vi "XXPathPlanner_Path_RePlan_Worker3.vi"(4 "StartingPoseTranslation":T1 {"Y" format="%14.3f"; "X" format="%14.3f"}, 5 "in PathPlannerPath":T2={"Reversed"=FALSE, "RotationTargets"=[], "ConstraintZones"=[], "EventMarkers"=[], "GlobalConstraints"={"MaxVelocityMps;"=0.0, "MaxAccelerationMpsSq;"=0.0, "MaxAngularVelRadPsEc;"=0.0, "MaxAngularAccRadPSecSq"=0.0, "Exists"=FALSE, "Unlimited"=FALSE, "NominalVoltageVolts"=12.0}, "GoalEndState"={"VelocityMPS"=0.0, "Rotation"={"VALUE"=0.0, "COS"=0.0, "SIN"=0.0}}, "AllPoints"=[], "Name"="", "Waypoints"=[], "PointTowardsZones"=[], "IdealStartingState"={"VelocityMPS"=0.0, "Rotation"={"VALUE"=0.0, "COS"=0.0, "SIN"=0.0}}, "IsChoreoPath"=FALSE, "PreventFlipping"=FALSE} {"IdealStartingState"."Rotation"."SIN" format="%13.4f"; "IdealStartingState"."Rotation"."COS" format="%13.4f"; "IdealStartingState"."Rotation"."VALUE" format="%13.4f"; "PointTowardsZones"."TargetPosition"."Y" format="%14.3f"; "PointTowardsZones"."TargetPosition"."X" format="%14.3f"; "PointTowardsZones"."RotationOffset"."SIN" format="%13.4f"; "PointTowardsZones"."RotationOffset"."COS" format="%13.4f"; "PointTowardsZones"."RotationOffset"."VALUE" format="%13.4f"; "Waypoints"."nextControl"."Y" format="%14.3f"; "Waypoints"."nextControl"."X" format="%14.3f"; "Waypoints"."anchor"."Y" format="%14.3f"; "Waypoints"."anchor"."X" format="%14.3f"; "Waypoints"."prevControl"."Y" format="%14.3f"; "Waypoints"."prevControl"."X" format="%14.3f"; "AllPoints"."RotationTarget"."rotation"."SIN" format="%13.4f"; "AllPoints"."RotationTarget"."rotation"."COS" format="%13.4f"; "AllPoints"."RotationTarget"."rotation"."VALUE" format="%13.4f"; "AllPoints"."Position"."Y" format="%14.3f"; "AllPoints"."Position"."X" format="%14.3f"; "GoalEndState"."Rotation"."SIN" format="%13.4f"; "GoalEndState"."Rotation"."COS" format="%13.4f"; "GoalEndState"."Rotation"."VALUE" format="%13.4f"; "RotationTargets"."rotation"."SIN" format="%13.4f"; "RotationTargets"."rotation"."COS" format="%13.4f"; "RotationTargets"."rotation"."VALUE" format="%13.4f"}, 6 "robotNextCtrl":T1 {"Y" format="%14.3f"; "X" format="%14.3f"}, 7 "NumPtsMinusOne":i32, 8 "ClosestPointIdx":i32, 9 "robotNextCtrl_NULL":bool, 11 "ClosestDist":dbl) -> (2 "Error":bool, 3 "Replanned Path":T2={"Reversed"=FALSE, "RotationTargets"=[], "ConstraintZones"=[], "EventMarkers"=[], "GlobalConstraints"={"MaxVelocityMps;"=0.0, "MaxAccelerationMpsSq;"=0.0, "MaxAngularVelRadPsEc;"=0.0, "MaxAngularAccRadPSecSq"=0.0, "Exists"=FALSE, "Unlimited"=FALSE, "NominalVoltageVolts"=12.0}, "GoalEndState"={"VelocityMPS"=0.0, "Rotation"={"VALUE"=0.0, "COS"=0.0, "SIN"=0.0}}, "AllPoints"=[], "Name"="", "Waypoints"=[], "PointTowardsZones"=[], "IdealStartingState"={"VelocityMPS"=0.0, "Rotation"={"VALUE"=0.0, "COS"=0.0, "SIN"=0.0}}, "IsChoreoPath"=FALSE, "PreventFlipping"=FALSE} {"IdealStartingState"."Rotation"."SIN" format="%13.4f"; "IdealStartingState"."Rotation"."COS" format="%13.4f"; "IdealStartingState"."Rotation"."VALUE" format="%13.4f"; "PointTowardsZones"."TargetPosition"."Y" format="%14.3f"; "PointTowardsZones"."TargetPosition"."X" format="%14.3f"; "PointTowardsZones"."RotationOffset"."SIN" format="%13.4f"; "PointTowardsZones"."RotationOffset"."COS" format="%13.4f"; "PointTowardsZones"."RotationOffset"."VALUE" format="%13.4f"; "Waypoints"."nextControl"."Y" format="%14.3f"; "Waypoints"."nextControl"."X" format="%14.3f"; "Waypoints"."anchor"."Y" format="%14.3f"; "Waypoints"."anchor"."X" format="%14.3f"; "Waypoints"."prevControl"."Y" format="%14.3f"; "Waypoints"."prevControl"."X" format="%14.3f"; "AllPoints"."RotationTarget"."rotation"."SIN" format="%13.4f"; "AllPoints"."RotationTarget"."rotation"."COS" format="%13.4f"; "AllPoints"."RotationTarget"."rotation"."VALUE" format="%13.4f"; "AllPoints"."Position"."Y" format="%14.3f"; "AllPoints"."Position"."X" format="%14.3f"; "GoalEndState"."Rotation"."SIN" format="%13.4f"; "GoalEndState"."Rotation"."COS" format="%13.4f"; "GoalEndState"."Rotation"."VALUE" format="%13.4f"; "RotationTargets"."rotation"."SIN" format="%13.4f"; "RotationTargets"."rotation"."COS" format="%13.4f"; "RotationTargets"."rotation"."VALUE" format="%13.4f"})   [LabVIEW 2019]
doc: "Replan path worker 3\n\nInternal routine. Not for end user use."
uses:
  PathPlanner24.lvlib
  <vilib>/Rock Robotics/WPI/ThirdParty/JAS_Junk/TrajLib/Trajectory_Library.lvlib
  <vilib>/Rock Robotics/WPI/ThirdParty/JAS_Junk/TrajLib/TypeDef/TRANSLATION2D.ctl
  <vilib>/Rock Robotics/WPI/ThirdParty/JAS_Junk/TrajLib/TypeDef/ROTATION2D.ctl
  TypeDef/PathPlannerRotationTarget.ctl
  TypeDef/PathPlannerPathConstraints.ctl
  TypeDef/PathPlannerConstraintsZone.ctl
  ENum/PathPlanner_CommandUtilType_ENUM.ctl
  TypeDef/PathPlannerCommandUtil.ctl
  TypeDef/PathPlannerEventMarker.ctl
  TypeDef/PathPlannerGoalEndState.ctl
  TypeDef/PathPlannerPathPoint.ctl
  TypeDef/PathPlannerPath.ctl
  TypeDef/PathPlannerWaypoint.ctl
  TypeDef/PathPlannerPointTowardsZone.ctl
  TypeDef/PathPlannerIdealStartingState.ctl
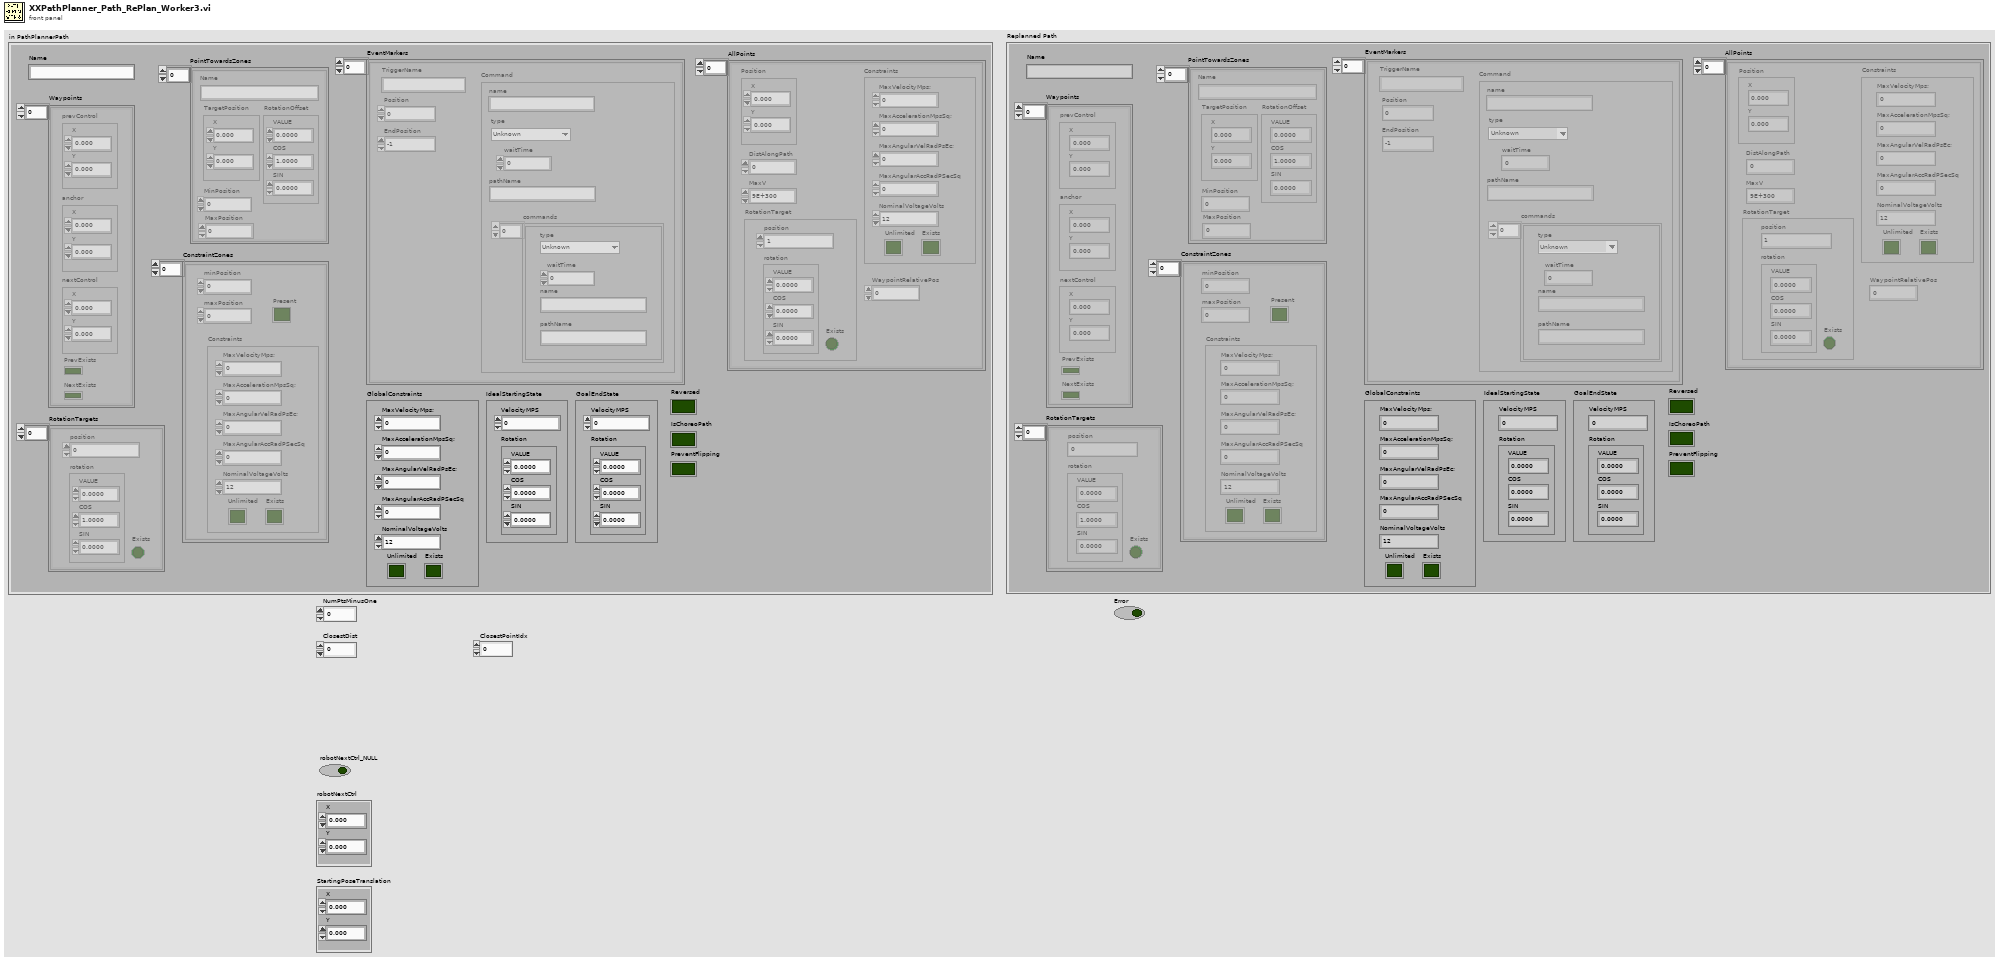
[diagram p1: front panel]
types:
  T1 = typedef "Trajectory_Library.lvlib/TRANSLATION2D.ctl" = cluster{"X":dbl, "Y":dbl}
  T2 = typedef "PathPlanner24.lvlib/PathPlannerPath.ctl" = cluster{"Reversed":bool, "RotationTargets":T3[], "ConstraintZones":T5[], "EventMarkers":T7[], "GlobalConstraints":T6, "GoalEndState":T10, "AllPoints":T11[], "Name":string, "Waypoints":T12[], "PointTowardsZones":T13[], "IdealStartingState":T14, "IsChoreoPath":bool, "PreventFlipping":bool}
  T3 = typedef "PathPlanner24.lvlib/PathPlannerRotationTarget.ctl" = cluster{"rotation":T4, "position":dbl, "Exists":bool}
  T4 = typedef "Trajectory_Library.lvlib/ROTATION2D.ctl" = cluster{"VALUE":dbl, "COS":dbl, "SIN":dbl}
  T5 = typedef "PathPlanner24.lvlib/PathPlannerConstraintsZone.ctl" = cluster{"minPosition":dbl, "maxPosition":dbl, "Constraints":T6, "Present":bool}
  T6 = typedef "PathPlanner24.lvlib/PathPlannerPathConstraints.ctl" = cluster{"MaxVelocityMps;":dbl, "MaxAccelerationMpsSq;":dbl, "MaxAngularVelRadPsEc;":dbl, "MaxAngularAccRadPSecSq":dbl, "Exists":bool, "Unlimited":bool, "NominalVoltageVolts":dbl}
  T7 = typedef "PathPlanner24.lvlib/PathPlannerEventMarker.ctl" = cluster{"Position":dbl, "Command":T8, "TriggerName":string, "EndPosition":dbl}
  T8 = typedef "PathPlanner24.lvlib/PathPlannerCommandUtil.ctl" = cluster{"waitTime":dbl, "name":string, "pathName":string, "commands":cluster{"type":T9, "waitTime":dbl, "name":string, "pathName":string}[], "type":T9}
  T9 = typedef "PathPlanner24.lvlib/PathPlanner_CommandUtilType_ENUM.ctl" = enum16{"Unknown", "Wait", "Named", "Path", "Sequential", "Parallel", "Race", "Deadline"}
  T10 = typedef "PathPlanner24.lvlib/PathPlannerGoalEndState.ctl" = cluster{"VelocityMPS":dbl, "Rotation":T4}
  T11 = typedef "PathPlanner24.lvlib/PathPlannerPathPoint.ctl" = cluster{"Position":T1, "DistAlongPath":dbl, "MaxV":dbl, "Constraints":T6, "RotationTarget":T3, "WaypointRelativePos":dbl}
  T12 = typedef "PathPlanner24.lvlib/PathPlannerWaypoint.ctl" = cluster{"prevControl":T1, "anchor":T1, "nextControl":T1, "PrevExists":bool, "NextExists":bool}
  T13 = typedef "PathPlanner24.lvlib/PathPlannerPointTowardsZone.ctl" = cluster{"RotationOffset":T4, "Name":string, "TargetPosition":T1, "MinPosition":dbl, "MaxPosition":dbl}
  T14 = typedef "PathPlanner24.lvlib/PathPlannerIdealStartingState.ctl" = cluster{"VelocityMPS":dbl, "Rotation":T4}
  T15 = typedef "PathPlannerPathSegment.ctl" = cluster{"SegmentPoints":T11[]}
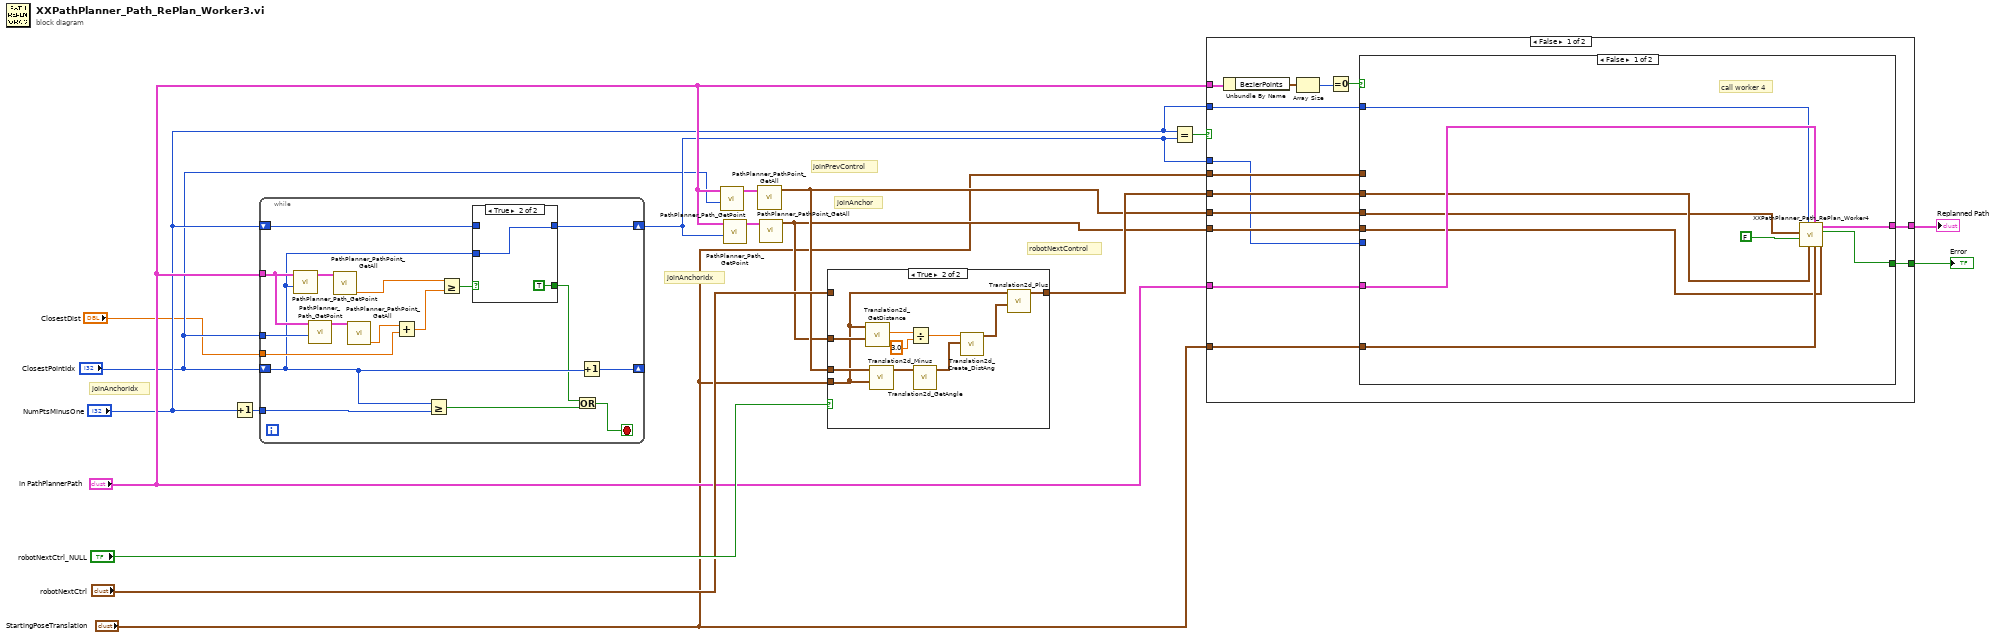
[diagram p0: block diagram]
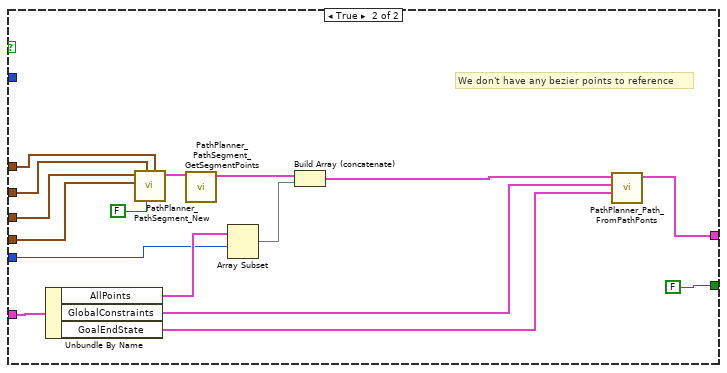
[diagram p2: hidden frame]
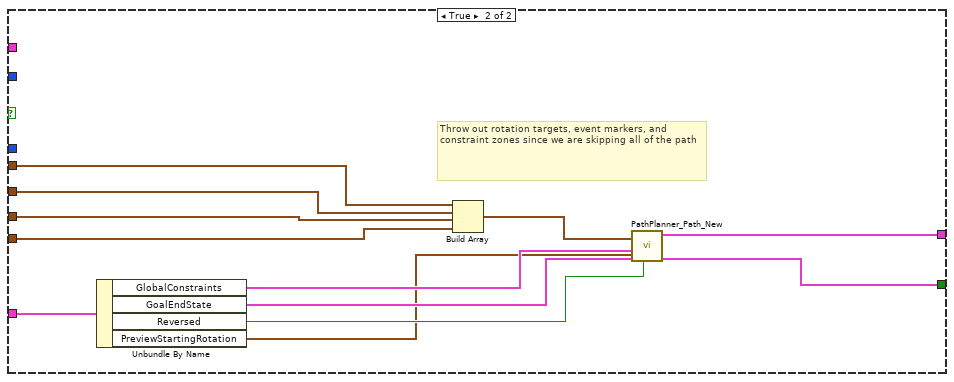
[diagram p3: hidden frame]
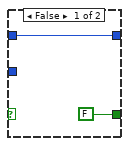
[diagram p5: hidden frame]
diagram:
  # "robotNextControl"
  # "joinAnchor"
  # "joinPrevControl"
  # "joinAnchorIdx"
  # "joinAnchorIdx"
  n1 = Increment(x="NumPtsMinusOne") -> (x+1=w17:i32)
  n2 = while {
    shift-right: [w33] -> _
    shift-left: "ClosestPointIdx" -> [w21]
    tunnel: w17 -> [w34]
    tunnel: "in PathPlannerPath" -> [w29]
    tunnel: "ClosestPointIdx" -> [w30]
    tunnel: "ClosestDist" -> [w27]
    shift-right: [w19] -> w5
    shift-left: "NumPtsMinusOne" -> [w20]
    stop <- w22 stop-if-true
    n3 = call "PathPlanner_Path_GetPoint.vi"("Index"=w21, "PathPlannerPath"=w29) -> ("Point"=w32:T11)  [unwired: 9 in]
    n4 = call "PathPlanner_Path_GetPoint.vi"("Index"=w30, "PathPlannerPath"=w29) -> ("Point"=w31:T11)  [unwired: 9 in]
    n5 = call "PathPlanner_PathPoint_GetAll.vi"("PathPlannerPoint"=w32) -> ("DistAlongPath"=w26:dbl)  [unwired: 5 in, 5 out]
    n6 = call "PathPlanner_PathPoint_GetAll.vi"("PathPlannerPoint"=w31) -> ("DistAlongPath"=w28:dbl)  [unwired: 5 in, 5 out]
    n7 = Add(x=w28, y=w27) -> (x+y=w25:dbl)
    n8 = Greater Or Equal?(x=w21, y=w34) -> (x >= y?=w23:bool)
    n9 = Greater Or Equal?(x=w26, y=w25) -> (x >= y?=w24:bool)
    n10 = case shown="True" w24 {
      tunnel: w21 -> [_ w38]
      tunnel: w20 -> [w36 _]
      tunnel: [w36 w38] -> w19
      tunnel: [FALSE TRUE] -> w18
      frame False {
      }
      frame True {
      }
    }
    n11 = Or(x=w18, y=w23) -> (x .or. y?=w22:bool)
    n12 = Increment(x=w21) -> (x+1=w33:i32)
  }
  n13 = call "PathPlanner_Path_GetPoint.vi"("Index"="ClosestPointIdx", "PathPlannerPath"="in PathPlannerPath") -> ("Point"=w16:T11)  [unwired: 9 in]
  n14 = call "PathPlanner_Path_GetPoint.vi"("Index"=w5, "PathPlannerPath"="in PathPlannerPath") -> ("Point"=w15:T11)  [unwired: 9 in]
  n15 = call "PathPlanner_PathPoint_GetAll.vi"("PathPlannerPoint"=w16) -> ("Position"=w10:T1)  [unwired: 5 in, 5 out]
  n16 = call "PathPlanner_PathPoint_GetAll.vi"("PathPlannerPoint"=w15) -> ("Position"=w9:T1)  [unwired: 5 in, 5 out]
  n17 = case shown="True" "robotNextCtrl_NULL" {
    tunnel: "robotNextCtrl" -> [w39 _]
    tunnel: [w39 w42] -> w11
    tunnel: w9 -> [_ w45]
    tunnel: w10 -> [_ w46]
    tunnel: "StartingPoseTranslation" -> [_ w44]
    frame False {
    }
    frame True {
      n18 = call <vilib>:"Translation2d_GetDistance.vi"("other Translation"=w45, "In Translation"=w44) -> ("Distance"=w48:dbl)  [unwired: 9 in]
      n19 = call <vilib>:"Translation2d_Minus.vi"("other Translation"=w44, "In Translation"=w46) -> ("Out Translation"=w49:T1)  [unwired: 9 in]
      n20 = Divide(x=w48, y=3.0) -> (x/y=w41:dbl)
      n21 = call <vilib>:"Translation2d_GetAngle.vi"("In Translation"=w49) -> ("Angle_Rotation2d"=w40:T4)  [unwired: 10 in]
      n22 = call <vilib>:"Translation2d_Create_DistAng.vi"("Angle"=w40, "Dist"=w41) -> ("TRANSLATION"=w43:T1)  [unwired: 9 in]
      n23 = call <vilib>:"Translation2d_Plus.vi"("other Translation"=w43, "In Translation"=w44) -> ("Out Translation"=w42:T1)  [unwired: 9 in]
    }
  }
  n24 = Equal?(x="NumPtsMinusOne", y=w5) -> (x = y?=w12:bool)
  n25 = case shown="False" w12 {
    tunnel: "StartingPoseTranslation" -> [w56 w100]
    tunnel: w11 -> [w55 w99]
    tunnel: w10 -> [w54 w98]
    tunnel: w9 -> [w53 w97]
    tunnel: "in PathPlannerPath" -> [w59 w95]
    tunnel: [w58 w90] -> w8
    tunnel: [w57 w89] -> w7
    tunnel: "in PathPlannerPath" -> [w63 _]
    tunnel: w5 -> [w52 _]
    tunnel: "NumPtsMinusOne" -> [w51 _]
    tunnel: "StartingPoseTranslation" -> [w50 _]
    frame False {
      n26 = Unbundle By Name(w63) -> ("BezierPoints"=w62:T1[])
      n27 = Array Size(array=w62) -> (size(s)=w61:i32)
      n28 = Equal To 0?(x=w61) -> (x = 0?=w60:bool)
      n29 = case shown="False" w60 {
        tunnel: w59 -> [w70 w88]
        tunnel: [w72 w74] -> w58
        tunnel: [w71 FALSE] -> w57
        tunnel: w56 -> [_ w87]
        tunnel: w55 -> [w67 w86]
        tunnel: w54 -> [w64 w85]
        tunnel: w53 -> [w65 w84]
        tunnel: w52 -> [_ w79]
        tunnel: w51 -> [w69 _]
        tunnel: w50 -> [w66 _]
        frame False {
          # "call worker 4"
          n30 = call "XXPathPlanner_Path_RePlan_Worker4.vi"("JoinAnchor"=w65, "StartingPoseTranslation"=w66, "in PathPlannerPath"=w70, "robotNextCtrl"=w67, "NumPtsMinusOne"=w69, "robotNextCtrl_NULL"=FALSE, "JoinPrevCtrl"=w64) -> ("Error"=w71:bool, "Replanned Path"=w72:T2)  [unwired: 3 in]
        }
        frame True {
          # "We don't have any bezier points to reference"
          n31 = Unbundle By Name(w88) -> ("AllPoints"=w80:T11[], "GlobalConstraints"=w76:T6, "GoalEndState"=w75:T10)
          n32 = call "PathPlanner_PathSegment_New.vi"("P1"=w87, "EndSegment"=FALSE, "P2"=w86, "P4"=w84, "P3"=w85) -> ("Segment"=w82:T15)  [unwired: 6 in]
          n33 = call "PathPlanner_PathSegment_GetSegmentPoints.vi"("Segment"=w82) -> ("SegmentPoints"=w81:T11[])  [unwired: 10 in]
          n34 = Array Subset(array=w80, index=w79) -> (w78:T11[])  [unwired: 1 in]
          n35 = Build Array (concatenate)(w81, w78) -> (w77:T11[])
          n36 = call "PathPlanner_Path_FromPathPonts.vi"("GoalEndState"=w75, "GlobalConstraints"=w76, "PathPoints"=w77) -> ("PathPlannerPath"=w74:T2)  [unwired: 8 in]
        }
      }
    }
    frame True {
      # "Throw out rotation targets, event markers, and constraint zones since we are skipping all of the path"
      n37 = Unbundle By Name(w95) -> ("GlobalConstraints"=w94:T6, "GoalEndState"=w93:T10, "Reversed"=w92:bool, "PreviewStartingRotation"=w91:T4)
      n38 = Build Array(w100, w99, w98, w97) -> (w96:T1[])
      n39 = call "PathPlanner_Path_New.vi"("IdealStartingState"=w91, "Waypoints"=w96, "Reversed"=w92, "GoalEndState"=w93, "GlobalConstraints"=w94) -> ("PointTowardsZones"=w89:T13[], "PathPlannerPath"=w90:T2)  [unwired: 4 in, 1 out]
    }
  }
  "Error" <- w7
  "Replanned Path" <- w8
